vi "yylltestresult Runner.vi"(7 "合格依据":T1, 8 "LowLimit-C":dbl, 9 "UpperLimit-B":dbl, 10 "StringLimit-A":string, 11 "DataIn-X":string) -> (1 "lowerLimit":string, 2 "upperLimit":string, 3 "isPass":bool)   [LabVIEW 2017]
uses:
  yylltestresult basis.ctl
  <vilib>/regexp/Match Regular Expression.xnode
panel:
  # "yylltestresult.Runner"
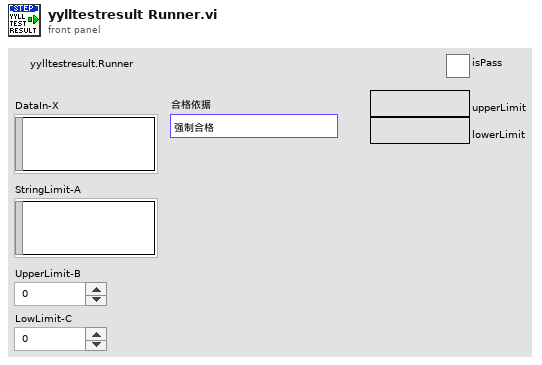
[diagram p1: front panel]
types:
  T1 = typedef "yylltestresult basis.ctl" = enum16{"强制合格", "强制不合格", "随机合格", "X=A", "X=\"真\"", "X=\"假\"", "X≠A", "X包含A", "X不包含A", "A包含X", "A包含非空X", "A不包含X", "X等于A正则匹配内容", "X包含A正则匹配内容", "X不包含A正则匹配内容", "X=B", "X≠B", "X＞B", "X≥B", "X＜B", "X≤B", "B≥X≥C", "B≥X＞C", "B＞X≥C", "B＞X＞C", "X≥B | C≥X", "X＞B | C≥X", "X≥B | C＞X", "X＞B | C＞X"}
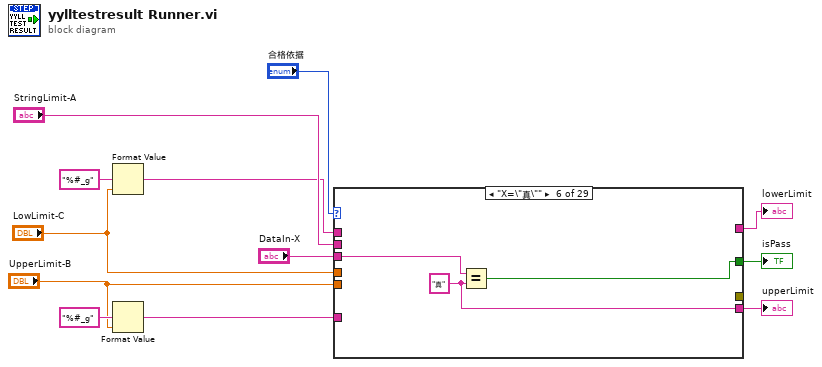
[diagram p0: block diagram]
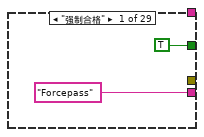
[diagram p2: hidden frame]
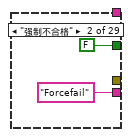
[diagram p3: hidden frame]
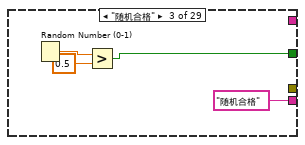
[diagram p4: hidden frame]
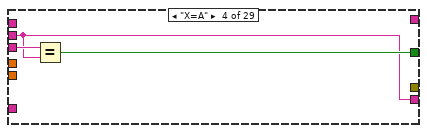
[diagram p5: hidden frame]
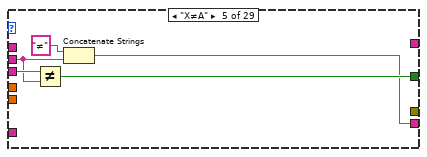
[diagram p6: hidden frame]
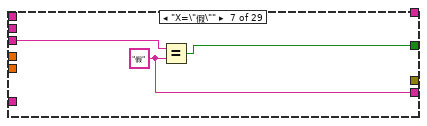
[diagram p7: hidden frame]
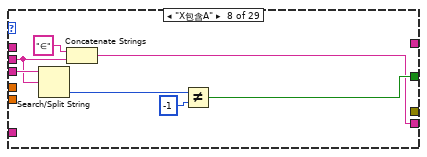
[diagram p8: hidden frame]
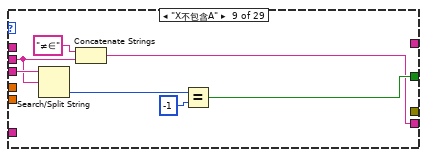
[diagram p9: hidden frame]
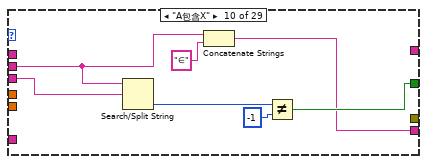
[diagram p10: hidden frame]
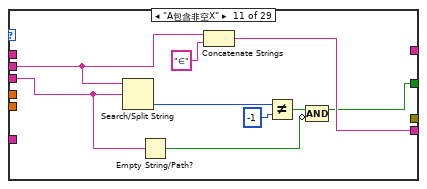
[diagram p11: hidden frame]
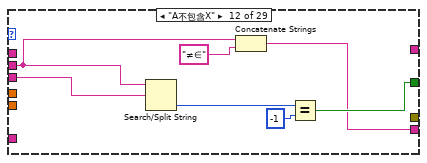
[diagram p12: hidden frame]
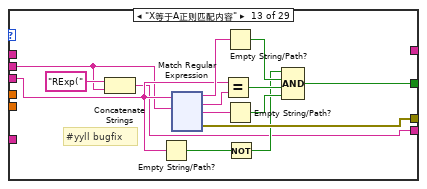
[diagram p13: hidden frame]
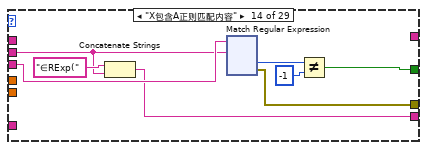
[diagram p14: hidden frame]
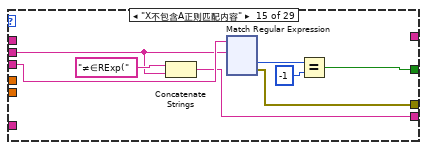
[diagram p15: hidden frame]
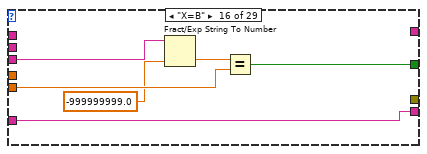
[diagram p16: hidden frame]
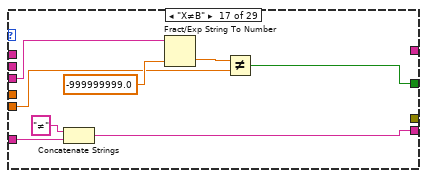
[diagram p17: hidden frame]
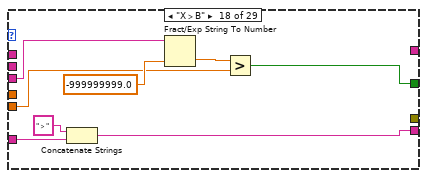
[diagram p18: hidden frame]
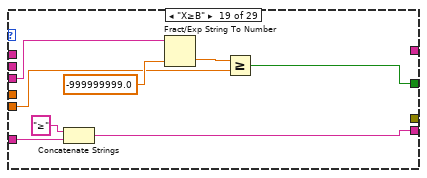
[diagram p19: hidden frame]
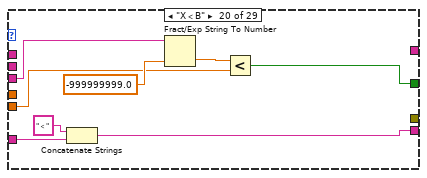
[diagram p20: hidden frame]
diagram:
  n1 = Format Value(format string="%#_g", value (0)="LowLimit-C") -> (output string=w2:string)  [unwired: 1 in]
  n2 = Format Value(format string="%#_g", value (0)="UpperLimit-B") -> (output string=w3:string)  [unwired: 1 in]
  n3 = case shown="\"X=\\\"真\\\"\"" "合格依据" {
    tunnel: [TRUE FALSE w17 w22 w27 w30 w33 w38 w45 w51 w57 w68 w78 w203 w325 w446 w453 w461 w469 w477 w485 w499 w511 w523 w535 w538 w555 w566 w580] -> w11
    tunnel: "DataIn-X" -> [_ _ _ w23 w28 w31 w34 w41 w46 w52 w58 w69 w77 w206 w328 w449 w455 w463 w471 w478 w487 w496 w508 w520 w532 w550 w564 w578 w592]
    tunnel: "StringLimit-A" -> [_ _ _ w21 w25 _ _ w36 w43 w50 w60 w66 w73 w201 w322 _ _ _ _ _ _ _ _ _ _ _ _ _ _]
    tunnel: "UpperLimit-B" -> [_ _ _ _ _ _ _ _ _ _ _ _ _ _ _ w447 w454 w462 w470 w479 w486 w498 w510 w522 w534 w543 w557 w571 w585]
    tunnel: "LowLimit-C" -> [_ _ _ _ _ _ _ _ _ _ _ _ _ _ _ _ _ _ _ _ _ w497 w509 w521 w533 w541 w553 w568 w583]
    tunnel: [_ _ _ _ _ _ _ _ _ _ _ _ w85 w207 w329 _ _ _ _ _ _ _ _ _ _ _ _ _ _] -> _
    tunnel: ["Forcepass" "Forcefail" "随机合格" w21 w24 w29 w32 w35 w42 w49 w59 w65 w72 w200 w323 w444 w450 w458 w466 w474 w482 w493 w504 w516 w527 w545 w559 w573 w587] -> w8
    tunnel: w3 -> [_ _ _ _ _ _ _ _ _ _ _ _ _ _ _ w444 w451 w459 w467 w475 w483 w494 w505 w517 w529 w547 w561 w575 w589]
    tunnel: w2 -> [_ _ _ _ _ _ _ _ _ _ _ _ _ _ _ _ _ _ _ _ _ w491 w503 w515 w528 w546 w560 w574 w588]
    tunnel: [_ _ _ _ _ _ _ _ _ _ _ _ _ _ _ _ _ _ _ _ _ w490 w502 w514 w526 w544 w558 w572 w586] -> w1
    frame "强制合格" {
    }
    frame "强制不合格" {
    }
    frame "随机合格" {
      n4 = Random Number (0-1)() -> (number: 0 to 1=w19:dbl)
      n5 = Greater?(x=w19, y=0.5) -> (0:w17:bool)
    }
    frame "X=A" {
      n6 = Equal?(x=w23, y=w21) -> (x = y?=w22:bool)
    }
    frame "X≠A" {
      n7 = Not Equal?(x=w28, y=w25) -> (x != y?=w27:bool)
      n8 = Concatenate Strings("≠" ("string"), w25) -> (w24:string)
    }
    frame "X=\"真\"" {
      w29 = "真" ("y")
      n9 = Equal?(x=w31, y=w29) -> (x = y?=w30:bool)
    }
    frame "X=\"假\"" {
      w32 = "假" ("y")
      n10 = Equal?(x=w34, y=w32) -> (x = y?=w33:bool)
    }
    frame "X包含A" {
      n11 = Search/Split String(string=w41, search string/char (-)=w36) -> (offset of match=w40:i32)  [unwired: 1 in, 2 out]
      n12 = Concatenate Strings("∈" ("string"), w36) -> (w35:string)
      n13 = Not Equal?(x=w40, y=-1) -> (x != y?=w38:bool)
    }
    frame "X不包含A" {
      n14 = Search/Split String(string=w46, search string/char (-)=w43) -> (offset of match=w48:i32)  [unwired: 1 in, 2 out]
      n15 = Concatenate Strings("≠∈" ("string"), w43) -> (w42:string)
      n16 = Equal?(x=w48, y=-1) -> (x = y?=w45:bool)
    }
    frame "A包含X" {
      n17 = Search/Split String(string=w50, search string/char (-)=w52) -> (offset of match=w55:i32)  [unwired: 1 in, 2 out]
      n18 = Concatenate Strings(w50, "∈" ("string")) -> (w49:string)
      n19 = Not Equal?(x=w55, y=-1) -> (x != y?=w51:bool)
    }
    frame "A包含非空X" {
      n20 = Search/Split String(string=w60, search string/char (-)=w58) -> (offset of match=w64:i32)  [unwired: 1 in, 2 out]
      n21 = Empty String/Path?(string/path=w58) -> (empty?=w56:bool)
      n22 = Concatenate Strings(w60, "∈" ("string")) -> (w59:string)
      n23 = Not Equal?(x=w64, y=-1) -> (x != y?=w61:bool)
      n24 = Compound Arithmetic op=AND(w61, invert w56) -> (w57:bool)
    }
    frame "A不包含X" {
      n25 = Search/Split String(string=w66, search string/char (-)=w69) -> (offset of match=w71:i32)  [unwired: 1 in, 2 out]
      n26 = Concatenate Strings(w66, "≠∈" ("string")) -> (w65:string)
      n27 = Equal?(x=w71, y=-1) -> (x = y?=w68:bool)
    }
    frame "X等于A正则匹配内容" {
      # "#yyll bugfix"
      n28 = Concatenate Strings("RExp(" ("string"), w73) -> (w72:string)
      n29 = Empty String/Path?(string/path=w77) -> (empty?=w76:bool)
      n30 = xnode "Match Regular Expression"("input string"=w77, "regular expression"=w73) -> ("before match"=w82:string, "whole match"=w84:string, "after match"=w81:string, "error out"=w85:errorcluster)  [unwired: 4 in, 1 out]
      n31 = Equal?(x=w77, y=w84) -> (x = y?=w83:bool)
      n32 = Empty String/Path?(string/path=w82) -> (empty?=w79:bool)
      n33 = Empty String/Path?(string/path=w81) -> (empty?=w80:bool)
      n34 = Not(x=w76) -> (.not. x?=w75:bool)
      n35 = Compound Arithmetic op=AND(w75, w79, w83, w80) -> (w78:bool)
    }
    frame "X包含A正则匹配内容" {
      n36 = Concatenate Strings("∈RExp(" ("string"), w201) -> (w200:string)
      n37 = xnode "Match Regular Expression"("input string"=w206, "regular expression"=w201) -> ("offset past match"=w205:i32, "error out"=w207:errorcluster)  [unwired: 4 in, 3 out]
      n38 = Not Equal?(x=w205, y=-1) -> (x != y?=w203:bool)
    }
    frame "X不包含A正则匹配内容" {
      n39 = Concatenate Strings("≠∈RExp(" ("string"), w322) -> (w323:string)
      n40 = xnode "Match Regular Expression"("input string"=w328, "regular expression"=w322) -> ("offset past match"=w327:i32, "error out"=w329:errorcluster)  [unwired: 4 in, 3 out]
      n41 = Equal?(x=w327, y=-1) -> (x = y?=w325:bool)
    }
    frame "X=B" {
      n42 = Fract/Exp String To Number(string=w449, default (0 dbl)=-999999999.0 ("default (0 DBL)")) -> (number=w448:dbl)  [unwired: 2 in, 1 out]
      n43 = Equal?(x=w448, y=w447) -> (x = y?=w446:bool)
    }
    frame "X≠B" {
      n44 = Concatenate Strings("≠" ("string"), w451) -> (w450:string)
      n45 = Fract/Exp String To Number(string=w455, default (0 dbl)=-999999999.0 ("default (0 DBL)")) -> (number=w457:dbl)  [unwired: 2 in, 1 out]
      n46 = Not Equal?(x=w457, y=w454) -> (x != y?=w453:bool)
    }
    frame "X＞B" {
      n47 = Concatenate Strings("＞" ("string"), w459) -> (w458:string)
      n48 = Fract/Exp String To Number(string=w463, default (0 dbl)=-999999999.0 ("default (0 DBL)")) -> (number=w465:dbl)  [unwired: 2 in, 1 out]
      n49 = Greater?(x=w465, y=w462) -> (0:w461:bool)
    }
    frame "X≥B" {
      n50 = Concatenate Strings("≥" ("string"), w467) -> (w466:string)
      n51 = Fract/Exp String To Number(string=w471, default (0 dbl)=-999999999.0 ("default (0 DBL)")) -> (number=w473:dbl)  [unwired: 2 in, 1 out]
      n52 = Greater Or Equal?(x=w473, y=w470) -> (x >= y?=w469:bool)
    }
    frame "X＜B" {
      n53 = Concatenate Strings("＜" ("string"), w475) -> (w474:string)
      n54 = Fract/Exp String To Number(string=w478, default (0 dbl)=-999999999.0 ("default (0 DBL)")) -> (number=w481:dbl)  [unwired: 2 in, 1 out]
      n55 = Less?(x=w481, y=w479) -> (x < y?=w477:bool)
    }
    frame "X≤B" {
      n56 = Concatenate Strings("≤" ("string"), w483) -> (w482:string)
      n57 = Fract/Exp String To Number(string=w487, default (0 dbl)=-999999999.0 ("default (0 DBL)")) -> (number=w489:dbl)  [unwired: 2 in, 1 out]
      n58 = Less Or Equal?(x=w489, y=w486) -> (x <= y?=w485:bool)
    }
    frame "B≥X≥C" {
      n59 = Concatenate Strings("≥" ("string"), w491) -> (w490:string)
      n60 = Concatenate Strings("≤" ("string"), w494) -> (w493:string)
      n61 = Fract/Exp String To Number(string=w496, default (0 dbl)=-999999999.0 ("default (0 DBL)")) -> (number=w500:dbl)  [unwired: 2 in, 1 out]
      n62 = In Range and Coerce(upper limit=w498, x=w500, lower limit=w497) -> (In Range?=w499:bool)  [unwired: 1 out]
    }
    frame "B≥X＞C" {
      n63 = Concatenate Strings("≤" ("string"), w505) -> (w504:string)
      n64 = Concatenate Strings("＞" ("string"), w503) -> (w502:string)
      n65 = Fract/Exp String To Number(string=w508, default (0 dbl)=-999999999.0 ("default (0 DBL)")) -> (number=w512:dbl)  [unwired: 2 in, 1 out]
      n66 = In Range and Coerce(upper limit=w510, x=w512, lower limit=w509) -> (In Range?=w511:bool)  [unwired: 1 out]
    }
    frame "B＞X≥C" {
      n67 = Concatenate Strings("≥" ("string"), w515) -> (w514:string)
      n68 = Concatenate Strings("＜" ("string"), w517) -> (w516:string)
      n69 = Fract/Exp String To Number(string=w520, default (0 dbl)=-999999999.0 ("default (0 DBL)")) -> (number=w524:dbl)  [unwired: 2 in, 1 out]
      n70 = In Range and Coerce(upper limit=w522, x=w524, lower limit=w521) -> (In Range?=w523:bool)  [unwired: 1 out]
    }
    frame "B＞X＞C" {
      n71 = Concatenate Strings("＞" ("string"), w528) -> (w526:string)
      n72 = Concatenate Strings("＜" ("string"), w529) -> (w527:string)
      n73 = Fract/Exp String To Number(string=w532, default (0 dbl)=-999999999.0 ("default (0 DBL)")) -> (number=w536:dbl)  [unwired: 2 in, 1 out]
      n74 = In Range and Coerce(upper limit=w534, x=w536, lower limit=w533) -> (In Range?=w535:bool)  [unwired: 1 out]
    }
    frame "X≥B | C≥X" {
      n75 = Concatenate Strings("≤" ("string"), w546) -> (w544:string)
      n76 = Concatenate Strings("≥" ("string"), w547) -> (w545:string)
      n77 = Fract/Exp String To Number(string=w550, default (0 dbl)=-999999999.0 ("default (0 DBL)")) -> (number=w542:dbl)  [unwired: 2 in, 1 out]
      n78 = Less Or Equal?(x=w542, y=w541) -> (x <= y?=w540:bool)
      n79 = Greater Or Equal?(x=w542, y=w543) -> (x >= y?=w539:bool)
      n80 = Or(x=w540, y=w539) -> (x .or. y?=w538:bool)
    }
    frame "X＞B | C≥X" {
      n81 = Concatenate Strings("≤" ("string"), w560) -> (w558:string)
      n82 = Concatenate Strings("＞" ("string"), w561) -> (w559:string)
      n83 = Fract/Exp String To Number(string=w564, default (0 dbl)=-999999999.0 ("default (0 DBL)")) -> (number=w554:dbl)  [unwired: 2 in, 1 out]
      n84 = Less Or Equal?(x=w554, y=w553) -> (x <= y?=w552:bool)
      n85 = Greater?(x=w554, y=w557) -> (0:w556:bool)
      n86 = Or(x=w552, y=w556) -> (x .or. y?=w555:bool)
    }
    frame "X≥B | C＞X" {
      n87 = Concatenate Strings("≥" ("string"), w575) -> (w573:string)
      n88 = Concatenate Strings("＜" ("string"), w574) -> (w572:string)
      n89 = Fract/Exp String To Number(string=w578, default (0 dbl)=-999999999.0 ("default (0 DBL)")) -> (number=w569:dbl)  [unwired: 2 in, 1 out]
      n90 = Less?(x=w569, y=w568) -> (x < y?=w567:bool)
      n91 = Greater Or Equal?(x=w569, y=w571) -> (x >= y?=w570:bool)
      n92 = Or(x=w567, y=w570) -> (x .or. y?=w566:bool)
    }
    frame "X＞B | C＞X" {
      n93 = Concatenate Strings("＜" ("string"), w588) -> (w586:string)
      n94 = Concatenate Strings("＞" ("string"), w589) -> (w587:string)
      n95 = Fract/Exp String To Number(string=w592, default (0 dbl)=-999999999.0 ("default (0 DBL)")) -> (number=w584:dbl)  [unwired: 2 in, 1 out]
      n96 = Less?(x=w584, y=w583) -> (x < y?=w582:bool)
      n97 = Greater?(x=w584, y=w585) -> (0:w581:bool)
      n98 = Or(x=w582, y=w581) -> (x .or. y?=w580:bool)
    }
  }
  "isPass" <- w11
  "upperLimit" <- w8
  "lowerLimit" <- w1
